vi "Read CCDF (Table).vi"(8 "error in (no error)":errorcluster, 11 "VISA resource name":refnum<visa-resource-name>) -> (0 "error out":errorcluster, 2 "CCDF Table Data":dbl[](array[numeric]), 3 "VISA resource name out":refnum<visa-resource-name>)   [LabVIEW 2018, in "Agilent U2000 Series.lvlib"]
doc: "Returns the data in CCDF table: average input power, probability at the average input power, peak-to-average power ratio, and sample count.\n\nNote:\nThis command is only applicable when the NORMal or DOUBle measurement speed setting is chosen.\nThis VI is not applicable for U2040 X-Series."
uses:
  Agilent U2000 Series.lvlib
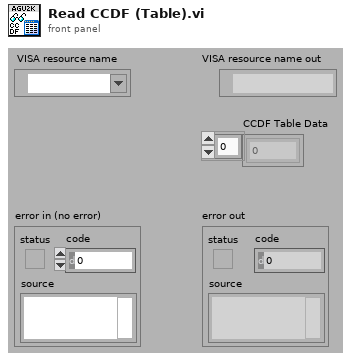
[diagram p1: front panel]
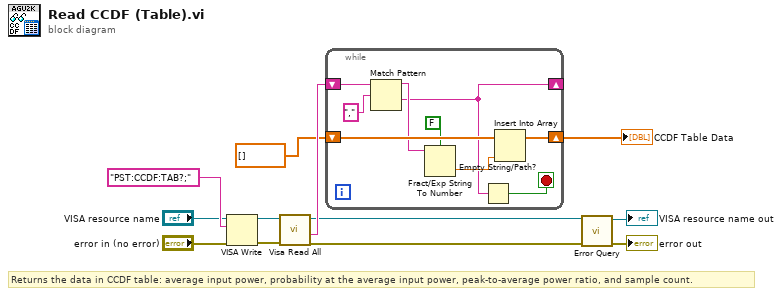
[diagram p0: block diagram]
diagram:
  # "Returns the data in CCDF table: average input power, probability at the average input power, peak-to-average power ratio, and sample count."
  n1 = VISA Write(VISA resource name="VISA resource name", write buffer="PST:CCDF:TAB?;", error in (no error)="error in (no error)") -> (VISA resource name out=w11:refnum<visa-resource-name>, error out=w10:errorcluster)  [unwired: 1 out]
  n2 = call "Visa Read All.vi"("error in (no error)"=w10, "VISA resource name"=w11) -> ("error out"=w1:errorcluster, "Read Buffer"=w9:string, "VISA resource name out"=w4:refnum<visa-resource-name>)  [unwired: 7 out]
  n3 = while {
    shift-right: [w14] -> _
    shift-left: w9 -> [w21]
    shift-right: [w17] -> w7
    shift-left: dbl[] [] -> [w19]
    stop <- w16 stop-if-true
    n4 = Match Pattern(string=w21, regular expression="," ("search string/char (-)")) -> (before substring=w15:string, after substring=w14:string)  [unwired: 3 out]
    n5 = Fract/Exp String To Number(use system decimal point (T)=FALSE, string=w15) -> (number=w18:dbl)  [unwired: 3 out]
    n6 = Empty String/Path?(string/path=w14) -> (empty?=w16:bool)
    n7 = Insert Into Array(array=w19, new element=w18) -> (w17:dbl[])  [unwired: 1 in]
  }
  "CCDF Table Data" <- w7
  n8 = call "Error Query.vi"("error in (no error)"=w1, "VISA resource name"=w4) -> ("error out"=→"error out":errorcluster, "VISA resource name out"=→"VISA resource name out":refnum<visa-resource-name>)  [unwired: 8 out]
